vi "Blue--constant.vi"() -> (1 "blue":u32)   [LabVIEW 2018, in "Resistor Band Colors.lvlib"]
uses:
  Resistor Band Colors.lvlib
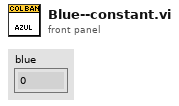
[diagram p1: front panel]
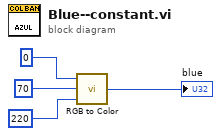
[diagram p0: block diagram]
diagram:
  n1 = call <vilib>:"RGB to Color.vi"("B"=u8 220 ("R"), "G"=u8 70 ("R"), "R"=u8 0) -> ("Color"=→"blue":u32)
